vi "Conversion Temperature.vi"(8 "error in (no error)":errorcluster, 11 "Service in":refnum<class "Service.lvclass">) -> (0 "error out":errorcluster, 3 "Service out":refnum<class "Service.lvclass">)   [LabVIEW 2021, in "Service.lvlib" / "Service.lvclass"]
uses:
  Service.lvclass
  Service.lvclass/Service.ctl
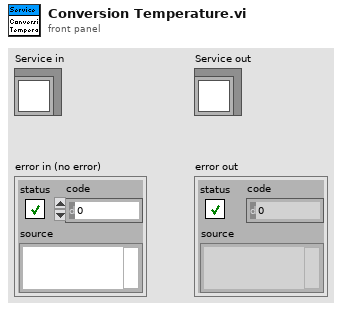
[diagram p1: front panel]
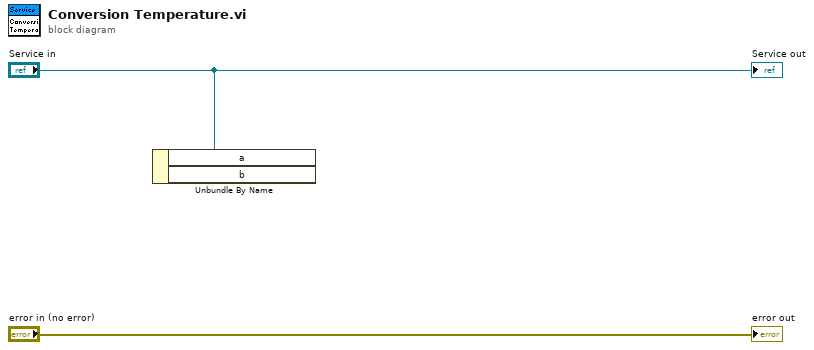
[diagram p0: block diagram]
diagram:
  n1 = Unbundle By Name("Service in") -> ()  [unwired: 2 out]
  "error out" <- "error in (no error)"
  "Service out" <- "Service in"
